vi "RichToFlatw4lvgrpc_Msg_ToServer_1.vi"(5 "OutputClusterType":T1, 11 "InputCluster":T2) -> (3 "OutputCluster":T1)   [LabVIEW 2019, in "Generated_server.lvlib"]
uses:
  Generated_server.lvlib
  w4lvgrpc_Msg_ToServer_1_Flat.ctl
  w4lvgrpc_Msg_ToServer_1.ctl
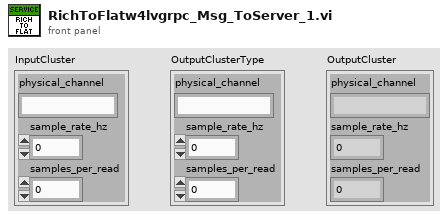
[diagram p1: front panel]
types:
  T1 = typedef "Generated_server.lvlib/w4lvgrpc_Msg_ToServer_1_Flat.ctl" = cluster{"physical_channel":string, "sample_rate_hz":dbl, "samples_per_read":i32}
  T2 = typedef "Generated_server.lvlib/w4lvgrpc_Msg_ToServer_1.ctl" = cluster{"physical_channel":string, "sample_rate_hz":dbl, "samples_per_read":i32}
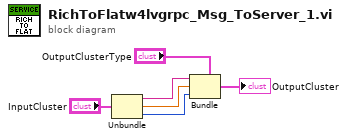
[diagram p0: block diagram]
diagram:
  n1 = Unbundle "Unbundle"("InputCluster") -> ("physical_channel"=w3:string, "sample_rate_hz"=w2:dbl, "samples_per_read"=w1:i32)
  n2 = Bundle "Bundle"(cluster="OutputClusterType", "physical_channel"=w3, "sample_rate_hz"=w2, "samples_per_read"=w1) -> (→"OutputCluster":T1)
